vi "Encode packed fixed32.vi"(7 "Field Number":i32, 10 "fixed32":u32[](array[numeric]), 11 "Buffer in":u8[](array[numeric]) format="%.0x") -> (3 "Buffer":u8[](array[numeric]) format="%.0x")   [LabVIEW 2020, in "LV-Proto.lvlib"]
uses:
  LV-Proto.lvlib
  Wire Type.ctl
  Wire Encode Varint I32.vi
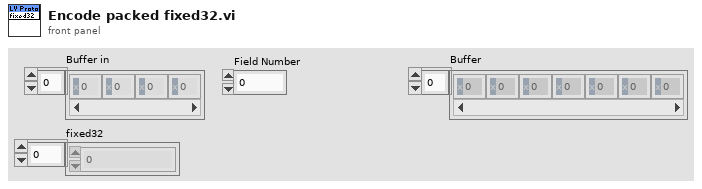
[diagram p1: front panel]
types:
  T1 = enum16{"big-endian, network order", "native, host order", "little-endian"}
  T2 = typedef "LV-Proto.lvlib/Wire Type.ctl" = enum8{"VARINT", "I64", "LEN", "SGROUP (Deprecated)", "EGROUP (Deprecated)", "I32"}
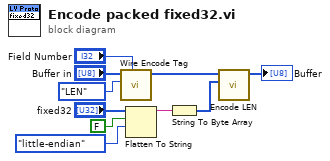
[diagram p0: block diagram]
diagram:
  n1 = call "Wire Encode Tag.vi"("Field Number"="Field Number", "Wire Type"=Wire_Type."LEN", "Buffer in"="Buffer in") -> ("Buffer"=w3:u8[])  [unwired: 8 in]
  n2 = Flatten To String(anything="fixed32", prepend array or string size? (T)=FALSE, byte order (0:big-endian, network order)=T1."little-endian") -> (data string=w6:string)  [unwired: 1 in, 2 out]
  n3 = String To Byte Array(string=w6) -> (unsigned byte array=w2:u8[])
  n4 = call "Encode LEN.vi"("Data"=w2, "Buffer in"=w3) -> ("Buffer"=→"Buffer":u8[])  [unwired: 9 in]
